vi "Get Transfer UIs.vi"(8 "error in":errorcluster, 11 "Component UI in":refnum<class "RDMA User Interfaces.lvclass">) -> (0 "error out":errorcluster, 1 "Tx Transfer UI":refnum<class "User Interface.lvclass">, 2 "Rx Transfer UI":refnum<class "User Interface.lvclass">, 3 "Component UI out":refnum<class "RDMA User Interfaces.lvclass">)   [LabVIEW 2020, in "RDMA.lvlib" / "RDMA User Interfaces.lvclass"]
uses:
  RDMA User Interfaces.lvclass
  DSF Core.lvlibp/Classes/User Interface/User Interface.lvclass
  RDMA User Interfaces.lvclass/RDMA User Interfaces.ctl
  Transfer Rx/RDMA Transfer Rx User Interface.lvclass
  Transfer Tx/RDMA Transfer Tx User Interface.lvclass
  C:/GitHub/rdma-plugin/Components/DSF Core.lvlibp/Classes/User Interface/User Interface.lvclass
  C:/GitHub/rdma-plugin/Components/Transceivers/RDMA/UI/Transfer Rx/RDMA Transfer Rx User Interface.lvclass
  C:/GitHub/rdma-plugin/Components/Transceivers/RDMA/UI/Transfer Tx/RDMA Transfer Tx User Interface.lvclass
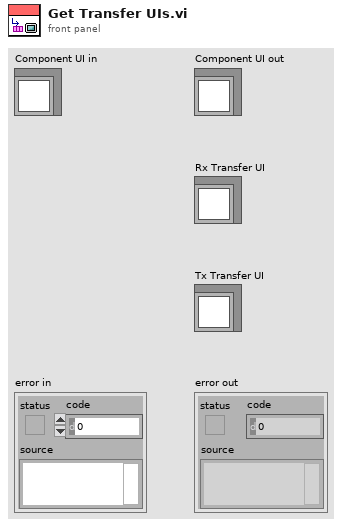
[diagram p1: front panel]
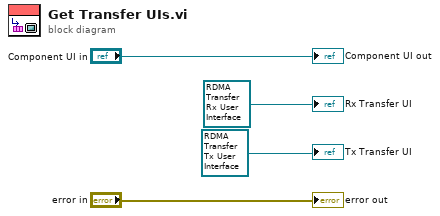
[diagram p0: block diagram]
diagram:
  "error out" <- "error in"
  "Component UI out" <- "Component UI in"
  "Rx Transfer UI" <- refnum<class "RDMA Transfer Rx User Interface.lvclass"> refnum ("RDMA.lvlib:RDMA Transfer Rx User Interface.lvclass")
  "Tx Transfer UI" <- refnum<class "RDMA Transfer Tx User Interface.lvclass"> refnum ("RDMA.lvlib:RDMA Transfer Tx User Interface.lvclass")
